vi "Get DQMH Modules.vi"(8 "error in":errorcluster, 10 "Include Dependencies":bool, 11 "Project in":refnum<class "Project.lvclass">) -> (0 "error out":errorcluster, 2 "DQMH Modules":T1[](array[typedef]), 3 "Project out":refnum<class "Project.lvclass">)   [LabVIEW 2019, in "Panther Dashboard.lvlib" / "Project.lvclass"]
uses:
  Project.lvclass
  <vilib>/Delacor/Delacor QMH/Libraries/Scripting API/Module Information--cluster.ctl
  Project.lvclass/Project.ctl
  Read Project Ref.vi
  Read Target Ref.vi
  <vilib>/Delacor/Delacor QMH/Libraries/Scripting API/DQMH_Scripting API.lvlib
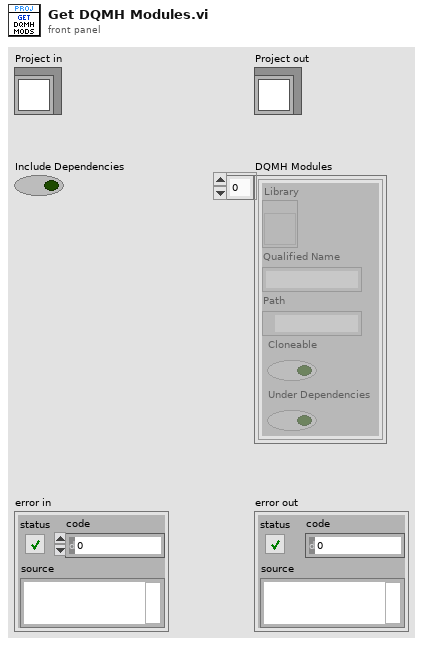
[diagram p1: front panel]
types:
  T1 = typedef "DQMH_Scripting API.lvlib/Module Information--cluster.ctl" = cluster{"Library":refnum<vi>, "Qualified Name":string, "Path":path, "Cloneable":bool, "Under Dependencies":bool}
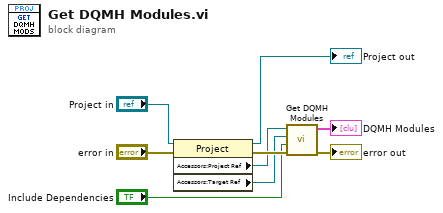
[diagram p0: block diagram]
diagram:
  n1 = property class="Project"(reference="Project in", error in="error in") -> (reference out=→"Project out":refnum<class "Project.lvclass">, error out=w9:errorcluster, "Accessors:Project Ref"=w5:refnum<vi>, "Accessors:Target Ref"=w6:refnum<vi>)
  n2 = call <vilib>:"Get DQMH Modules.vi"("error in"=w9, "Include Dependencies (F)"="Include Dependencies", "Target (My Computer)"=w6, "Project"=w5) -> ("error out"=→"error out":errorcluster, "DQMH Modules"=→"DQMH Modules":T1[])  [unwired: 6 in]
